vi "Dispenser_vac.vi"() -> ()   [LabVIEW 2016]
uses:
  <vilib>/Utility/file.llb/Read Delimited Spreadsheet (string).vi
  Other Models/EFD Ultimus V/EFD Ultimus V.lvlib
panel:
  in  "Pressure":dbl[](array[numeric])=[27.0, 27.0, 27.0, 27.0]
  out "Time(ms)":dbl
  out "Speed":dbl format="%#_13g"
  out "Comm":string
  in  "VISA resource name":refnum<visa-resource-name>="COM5"
  in  "Serial Configuration":T1={"Baud Rate "=115200, "Parity "=0, "Data Bits "=8, "Stop Bits"=10} {"Stop Bits" items=["1.0"=10, "1.5"=15, "2.0"=20]; "Data Bits" items=["7"=7, "8"=8]; "Parity" items=["None", "Odd", "Even"]; "Baud Rate" items=["9600"=9600, "19200"=19200, "38400"=38400, "115200"=115200]}
  in  "Z":dbl=58.56688 format="%#_13g"
  in  "Y":dbl=842.91108 format="%#_13g"
  in  "X":dbl=458.05353 format="%#_13g"
  in  "Path":path=path "C:/Users/TTUHEP/Documents/LabVIEW/Pattern/Pattern_sharpCorner_20200229_VaccumTEST.ngc"
  # "Origin"
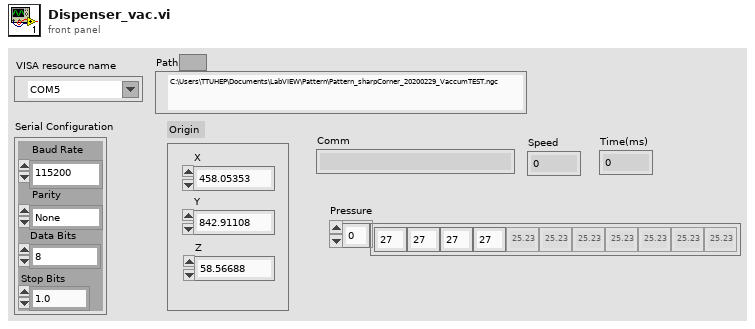
[diagram p1: front panel]
types:
  T1 = cluster{"Baud Rate ":u32, "Parity ":u16, "Data Bits ":u16, "Stop Bits":u16}
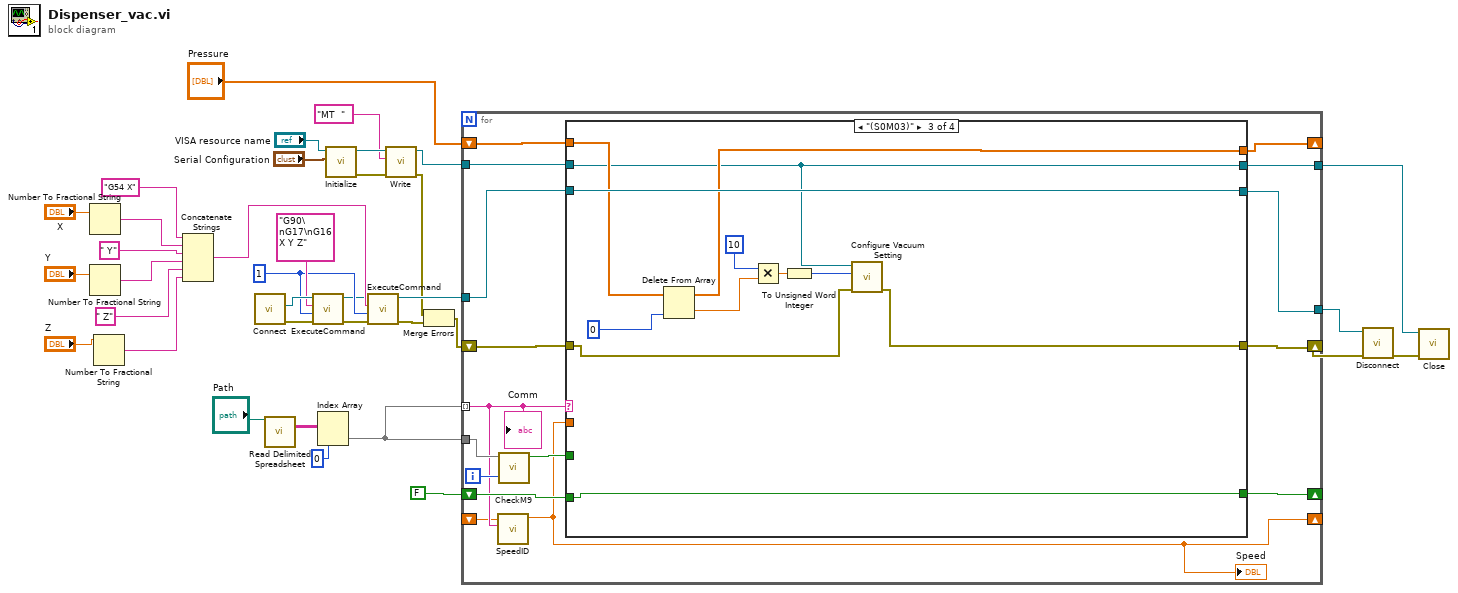
[diagram p0: block diagram]
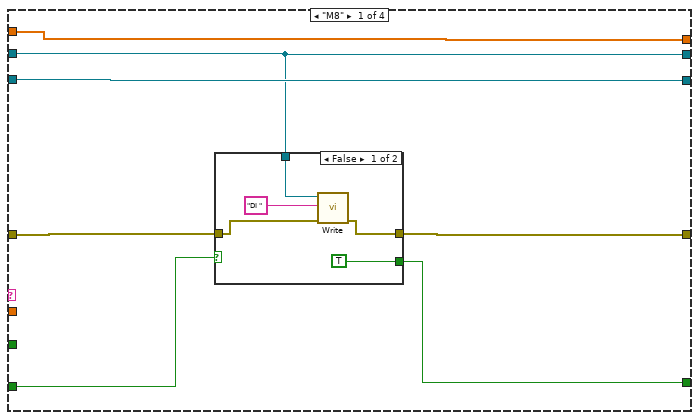
[diagram p2: hidden frame]
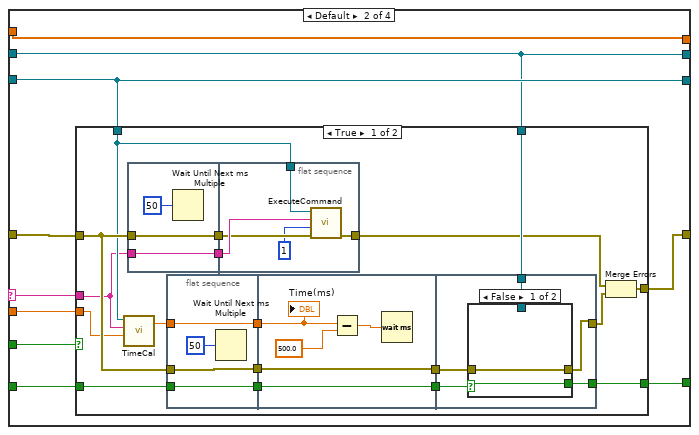
[diagram p4: hidden frame]
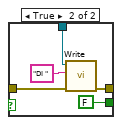
[diagram p5: hidden frame]
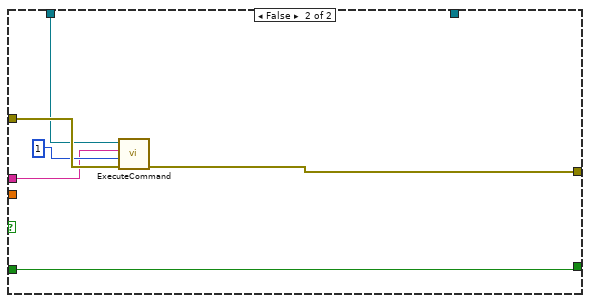
[diagram p6: hidden frame]
diagram:
  w4 = 1
  n1 = Number To Fractional String(number="X") -> (F-format string=w16:string)  [unwired: 3 in]
  n2 = Number To Fractional String(number="Y") -> (F-format string=w18:string)  [unwired: 3 in]
  n3 = Number To Fractional String(number="Z") -> (F-format string=w20:string)  [unwired: 3 in]
  n4 = Concatenate Strings("G54 X", w16, " Y", w18, " Z", w20) -> (w14:string)
  n5 = call "Connect.vi"() -> ("error out"=w2:errorcluster, "controller"=w13:refnum<k24>)  [unwired: 10 in]
  n6 = call-poly <vilib>:"Read Delimited Spreadsheet.vi"("file path (dialog if empty)"="Path") -> ("all rows"=w34:string[][])  [unwired: 9 in, 5 out]
  n7 = call "ExecuteCommand.vi"("taskId"=w4, "Command Code"="G90\nG17\nG16 X Y Z", "controller in"=w13) -> ("controller out"=w3:refnum<k24>)  [unwired: 6 in, 2 out]
  n8 = Index Array(array=w34, index (col)=0) -> (element=w6:string[])  [unwired: 1 in]
  n9 = call "Initialize.vi"("Serial Configuration"="Serial Configuration", "VISA resource name"="VISA resource name") -> ("error out"=w10:errorcluster, "VISA resource name out"=w9:refnum<visa-resource-name>)  [unwired: 8 in]
  n10 = call "ExecuteCommand.vi"("error in (no error)"=w2, "taskId"=w4, "Command Code"=w14, "controller in"=w3) -> ("error out"=w28:errorcluster, "controller out"=w31:refnum<k24>)  [unwired: 5 in, 1 out]
  n11 = call "Write.vi"("error in (no error)"=w10, "Command To Write"="MT  ", "VISA resource name"=w9) -> ("error out"=w7:errorcluster, "VISA resource name out"=w11:refnum<visa-resource-name>)  [unwired: 7 in]
  n12 = Merge Errors(w7, w28) -> (w27:errorcluster)
  n13 = for {
    tunnel: w6 -> [w41] mode=indexing
    shift-right: [w38] -> w26
    shift-left: w27 -> [w47]
    shift-right: [w49] -> _
    shift-left: FALSE -> [w50]
    tunnel: w31 -> [w48]
    tunnel: [w51] -> w5
    tunnel: w11 -> [w46]
    tunnel: [w45] -> w24
    tunnel: w6 -> [w44]
    shift-right: [w39] -> _
    shift-left: _ -> [w40]
    shift-right: [w36] -> _
    shift-left: "Pressure" -> [w37]
    i -> [w43]
    n14 = call "SpeedID.vi"("String"=w41, "Speed In"=w40) -> ("Speed Out"=w39:dbl)  [unwired: 9 in]
    "Speed" <- w39
    n15 = call "CheckM9.vi"("Index"=w43, "Comm list"=w44) -> ("Gonna Stop Next"=w42:bool)  [unwired: 9 in]
    n16 = case shown="\"(S0M03)\"" w41 {
      selector: w41 -> [_ w73 _ _]
      tunnel: w47 -> [w53 w75 w130 w144]
      tunnel: w48 -> [w58 w74 w140 w142]
      tunnel: [w57 w67 w129 w144] -> w38
      tunnel: [w58 w74 w140 w142] -> w51
      tunnel: w50 -> [w56 w71 w139 w145]
      tunnel: [w55 w70 w139 w145] -> w49
      tunnel: w46 -> [w54 w72 w132 w143]
      tunnel: [w54 w72 w132 w143] -> w45
      tunnel: w42 -> [_ w69 _ _]
      tunnel: w39 -> [_ w68 _ _]
      tunnel: w37 -> [w52 w66 w137 w141]
      tunnel: [w52 w66 w135 w141] -> w36
      frame "M8" {
        n17 = case shown="False" w56 {
          selector: w56 -> [_ w64]
          tunnel: w53 -> [w61 w65]
          tunnel: [w60 w65] -> w57
          tunnel: [TRUE w64] -> w55
          tunnel: w54 -> [w62 _]
          frame False {
            n18 = call "Write.vi"("error in (no error)"=w61, "Command To Write"="DI ", "VISA resource name"=w62) -> ("error out"=w60:errorcluster)  [unwired: 7 in, 1 out]
          }
          frame True {
          }
        }
      }
      frame Default {
        n19 = case shown="True" w69 {
          tunnel: w75 -> [w85 w128]
          tunnel: [w83 w127] -> w67
          tunnel: w74 -> [w78 w125]
          tunnel: w73 -> [w77 w124]
          tunnel: w72 -> [w91 _]
          tunnel: w71 -> [w93 w123]
          tunnel: [w92 w123] -> w70
          tunnel: w68 -> [w76 _]
          frame True {
            n20 = call "TimeCal.vi"("Speed In"=w76, "Command"=w77, "controller in"=w78) -> ("Time(ms)"=w79:dbl)  [unwired: 7 in, 1 out]
            n21 = flat-sequence {
              tunnel: w77 -> [w116]
              tunnel: [w116] -> w86
              tunnel: w85 -> [w115]
              tunnel: [w115] -> w84
              tunnel: w86 -> [w122]
              tunnel: w84 -> [w121]
              tunnel: [w120] -> w81
              tunnel: w78 -> [w119]
              frame #0 {
                n22 = Wait Until Next ms Multiple(millisecond multiple=50) -> ()  [unwired: 1 out]
              }
              frame #1 {
                n23 = call "ExecuteCommand.vi"("error in (no error)"=w121, "taskId"=1, "Command Code"=w122, "controller in"=w119) -> ("error out"=w120:errorcluster)  [unwired: 5 in, 2 out]
              }
            }
            n24 = flat-sequence {
              tunnel: w93 -> [w97]
              tunnel: [w97] -> w89
              tunnel: [w95] -> w88
              tunnel: w85 -> [w95]
              tunnel: w79 -> [w94]
              tunnel: [w94] -> w80
              tunnel: [w102] -> w90
              tunnel: w89 -> [w102]
              tunnel: w88 -> [w101]
              tunnel: [w101] -> w87
              tunnel: w80 -> [w99]
              tunnel: [w106] -> w92
              tunnel: [w105] -> w82
              tunnel: w91 -> [w104]
              tunnel: w90 -> [w107]
              tunnel: w87 -> [w103]
              frame #0 {
                n25 = Wait Until Next ms Multiple(millisecond multiple=50) -> ()  [unwired: 1 out]
              }
              frame #1 {
                n26 = Subtract(x=w99, y=500.0) -> (x-y=w100:dbl)
                n27 = Wait (ms)(milliseconds to wait=w100) -> ()  [unwired: 1 out]
                "Time(ms)" <- w99
              }
              frame #2 {
                n28 = case shown="False" w107 {
                  selector: w107 -> [w108 _]
                  tunnel: w103 -> [w109 w113]
                  tunnel: [w109 w112] -> w105
                  tunnel: [w108 FALSE] -> w106
                  tunnel: w104 -> [_ w111]
                  frame False {
                  }
                  frame True {
                    n29 = call "Write.vi"("error in (no error)"=w113, "Command To Write"="DI ", "VISA resource name"=w111) -> ("error out"=w112:errorcluster)  [unwired: 7 in, 1 out]
                  }
                }
              }
            }
            n30 = Merge Errors(w81, w82) -> (w83:errorcluster)
          }
          frame False {
            n31 = call "ExecuteCommand.vi"("error in (no error)"=w128, "taskId"=1, "Command Code"=w124, "controller in"=w125) -> ("error out"=w127:errorcluster)  [unwired: 5 in, 2 out]
          }
        }
      }
      frame "(S0M03)" {
        n32 = Delete From Array(array=w137, index=0) -> (deleted portion=w134:dbl, array with subset deleted=w135:dbl[])  [unwired: 1 in]
        n33 = Multiply(x=10, y=w134) -> (x*y=w133:dbl)
        n34 = To Unsigned Word Integer(number=w133) -> (unsigned 16bit integer=w131:u16)
        n35 = call "Configure Vacuum Setting.vi"("error in (no error)"=w130, "Vacuum Setting (0000)"=w131, "VISA resource name"=w132) -> ("error out"=w129:errorcluster)  [unwired: 7 in, 1 out]
      }
      frame "M9" {
      }
    }
    "Comm" <- w41
  }
  n36 = call "Disconnect.vi"("error in (no error)"=w26, "controller"=w5) -> ("error out"=w25:errorcluster)  [unwired: 9 in]
  n37 = call "Close.vi"("error in (no error)"=w25, "VISA resource name"=w24) -> ()  [unwired: 9 in, 1 out]
